vi "Autosize_Columns1.vi"() -> ()   [LabVIEW 2021]
panel:
  in  "Multicolumn Listbox":i32(listbox)
  # "Run the VI. The columns will autosize to fit the cell with the largest\nwidth. Note that this only works for 13pt font!"
  # "https://forums.ni.com/t5/LabVIEW/How-do-you-autosize-column-widths-in-a-multicolumn-listbox/td-p/31861"
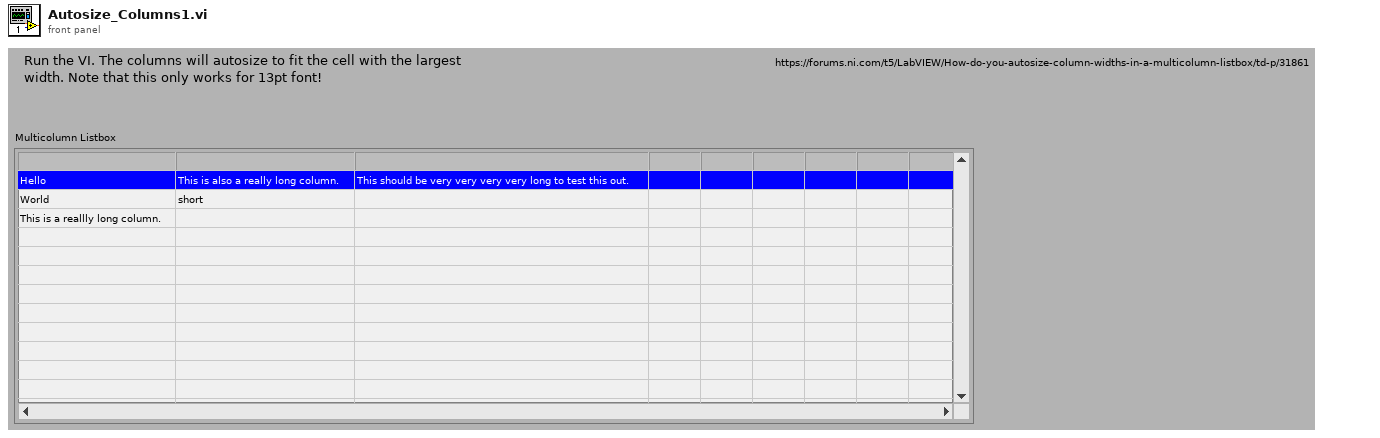
[diagram p1: front panel]
types:
  T1 = cluster{"left":i16, "top":i16, "right":i16, "bottom":i16}
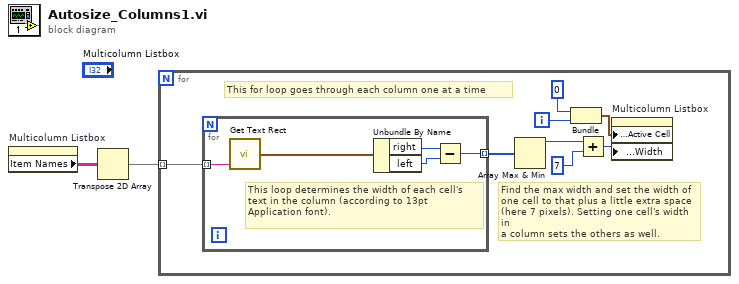
[diagram p0: block diagram]
diagram:
  n1 = property on="Multicolumn Listbox" class="MCListbox (strict)"() -> ("Item Names"=w2:string[][])  [unwired: 2 in, 2 out]
  n2 = Transpose 2D Array(2D array=w2) -> (transposed array=w1:string[][])
  n3 = for {
    tunnel: w1 -> [w10] mode=indexing
    i -> [w5]
    # "Find the max width and set the width of one cell to that plus a little extra space (here 7 pixels). Setting one cell's width in\na column sets the others as well."
    # "This for loop goes through each column one at a time"
    n4 = for {
      tunnel: w10 -> [w15] mode=indexing
      tunnel: [w11] -> w9 mode=indexing
      # "This loop determines the width of each cell's\ntext in the column (according to 13pt\nApplication font)."
      n5 = call <vilib>:"Get Text Rect.vi"("text"=w15) -> ("rect"=w14:T1)  [unwired: 8 in]
      n6 = Unbundle By Name(w14) -> ("right"=w13:i16, "left"=w12:i16)
      n7 = Subtract(x=w13, y=w12) -> (x-y=w11:i16)
    }
    n8 = Array Max & Min(array=w9) -> (max value=w3:i16)  [unwired: 3 out]
    n9 = Bundle(0, w5) -> (w4:cluster{i32, i32})  [unwired: 1 in]
    n10 = Add(x=w3, y=i16 7) -> (x+y=w6:i16)
    n11 = property on="Multicolumn Listbox" class="MCListbox (strict)"("Active Cell:Active Cell"=w4, "Active Cell:Cell Size:Width"=w6) -> ()  [unwired: 2 in, 2 out]
  }
